vi "getSweepResults.vi"(8 "error in (no error)":errorcluster, 11 "Instrument.LockinAPI in":refnum<class "Instrument.LockinAPI.lvclass">) -> (0 "error out":errorcluster, 1 "Y Results":waveform(dbl)[](array[waveform]), 2 "X results":waveform(dbl)[](array[waveform]), 3 "Instrument.LockinAPI out":refnum<class "Instrument.LockinAPI.lvclass">)   [LabVIEW 2019, in "Instrument.LockinAPI.lvclass"]
doc: "API to get the (sweep) results of lockin calculation.\n\nIf address=\"\", this API reads from localhost\nIf address is remote lockin, you need to add this computer to allowed whitelist on the lockin computer you are trying to access."
uses:
  Instrument.LockinAPI.lvclass
  Typedefs/LockinAPI.Commands--Enum.ctl
  Typedefs/LockinAPI.SweepData--Cluster.ctl
  6d578880-aa48-42d5-8634-c98e89a69395.vi
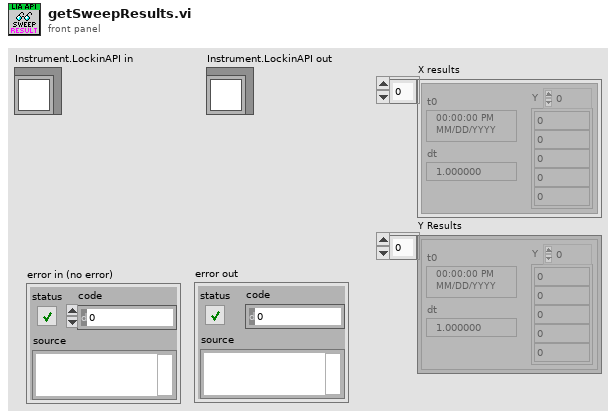
[diagram p1: front panel]
types:
  T1 = typedef "Instrument.LockinAPI.lvclass/LockinAPI.SweepData--Cluster.ctl" = cluster{"AO":waveform(dbl)[], "AI":waveform(dbl)[], "Xresults":waveform(dbl)[], "Yresults":waveform(dbl)[]}
  T2 = typedef "Instrument.LockinAPI.lvclass/LockinAPI.commands--Enum.ctl" = enum16{"setAI", "setAO", "setAO_Amplitude", "setAO_DC", "setAO_Frequency", "setAO_Phase", "setAO_Function", "setAO_I+", "setREF", "setREF_Frequency", "setREF_Phase", "setREF_TC", "setREF_Roll-Off", "setDAQ", "setSampling", "setOffset", "setState", "getState", "getAO", "getAI", "getResults", "getSampling", "getAOconfig", "getREFconfig", "setInputGain", "setOutputGain", "getInputGain", "getOutputGain", "setSamplingMode", "getSamplingMode", "setSweep", "setSweepTime", "setSweepTable", "getStatus", "getSweepResults", "getSweepWaveforms", "startSweep", "stopSweep", "setAUX", "getAUX"}
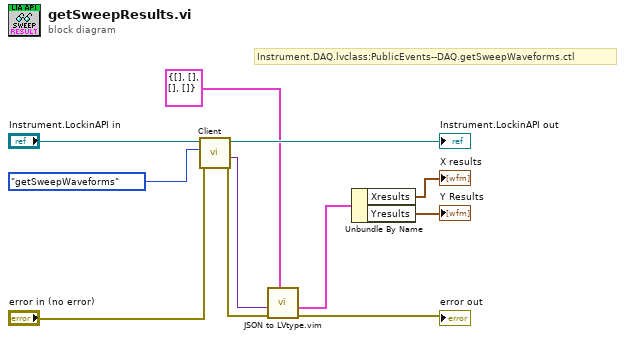
[diagram p0: block diagram]
diagram:
  # "Instrument.DAQ.lvclass:PublicEvents--DAQ.getSweepWaveforms.ctl"
  n1 = call-dynamic "Client.vi"("error in (no error)"="error in (no error)", "Command in"=LockinAPI.commands--Enum."getSweepWaveforms" ("Command"), "Instrument in"="Instrument.LockinAPI in") -> ("error out"=w4:errorcluster, "Data out"=w3:variant, "Instrument out"=→"Instrument.LockinAPI out":refnum<class "Instrument.LockinAPI.lvclass">)  [unwired: 5 in, 1 out]
  n2 = call "JSON to LVtype.vim"("type"=T1 {"AO"=[], "AI"=[], "Xresults"=[], "Yresults"=[]} ("sweepData"), "error in (no error)"=w4, "JSON Data in"=w3) -> ("error out"=→"error out":errorcluster, "Data out"=w5:T1)  [unwired: 7 in]
  n3 = Unbundle By Name(w5) -> ("Xresults"=→"X results":waveform(dbl)[], "Yresults"=→"Y Results":waveform(dbl)[])
